vi "Read Name.vi"(8 "error in (no error)":errorcluster, 11 "ARN":refnum<class "ARN.lvclass">) -> (0 "error out":errorcluster, 2 "Name":string, 3 "ARN out":refnum<class "ARN.lvclass">)   [LabVIEW 2015, in "NI_AWS_Core.lvlib" / "ARN.lvclass"]
uses:
  ARN.lvclass
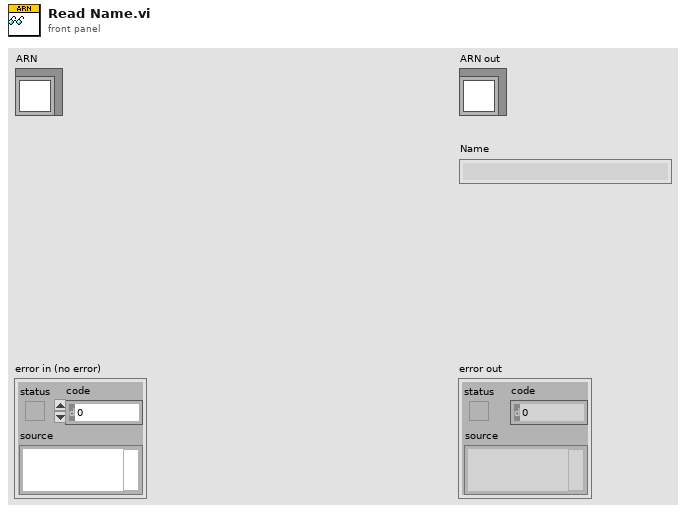
[diagram p1: front panel]
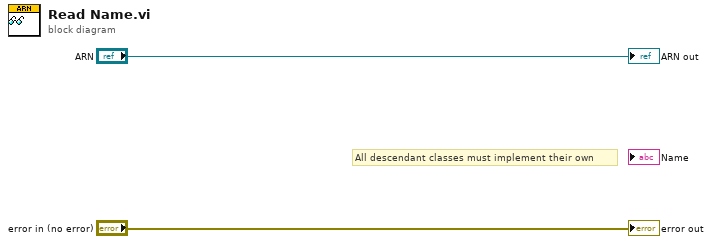
[diagram p0: block diagram]
diagram:
  # "All descendant classes must implement their own"
  "error out" <- "error in (no error)"
  "ARN out" <- "ARN"
